vi "CSDB_SVEdit.save SV CSV file.vi"(1 "CSVPath":path, 2 "SVHeader":string[](array[string]), 3 "SVValues":string[][](array[string]), 5 "error in":errorcluster) -> (19 "error out":errorcluster)   [LabVIEW 2014, in "CSDB_SVEdit.lvlib"]
doc: "Saves the header and the values of a Shared Variable configuration to a CSV file."
uses:
  CSDB_SVEdit.lvlib
  CSlibraries/UtilityLib/UtilityLib.lvlib
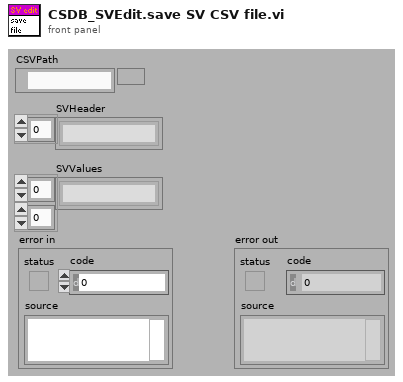
[diagram p1: front panel]
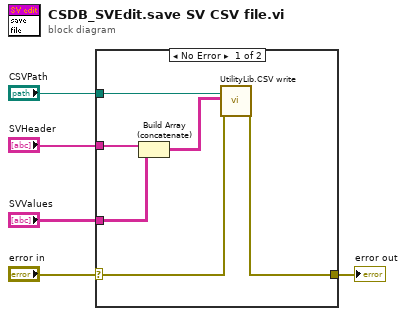
[diagram p0: block diagram]
diagram:
  n1 = case shown="No Error" "error in" {
    selector: "error in" -> [w6 w12]
    tunnel: "CSVPath" -> [w11 _]
    tunnel: "SVHeader" -> [w10 _]
    tunnel: "SVValues" -> [w9 _]
    tunnel: [w7 w12] -> w2
    frame No Error {
      n2 = Build Array (concatenate)(w10, w9) -> (w8:string[][])
      n3 = call "UtilityLib.CSV write.vi"("file (use dialog)"=w11, "CSVArray"=w8, "error in"=w6) -> ("error out"=w7:errorcluster)  [unwired: 16 in]
    }
    frame Error {
    }
  }
  "error out" <- w2
